vi "Arm Motor Control.vi"(6 "Left Arm EncoderDevRef":T1={"DevStatus"={"status"=FALSE, "code"=0, "source"=""}, "EncoderIndex"=enum."Invalid", "CounterIndex"=enum."Ctr 1", "DistancePerCount"=2.0, "Decoding Type"=enum."4x"}, 7 "Right Arm EncoderDevRef":T1={"DevStatus"={"status"=FALSE, "code"=0, "source"=""}, "EncoderIndex"=enum."Invalid", "CounterIndex"=enum."Ctr 1", "DistancePerCount"=2.0, "Decoding Type"=enum."4x"}, 8 "Right Arm MotorControlDevRef":T5={"DeviceStatus"={"status"=FALSE, "code"=0, "source"=""}, "Type"=enum."PWM", "PWM"={"PWM Channel"=enum."Invalid", "DeadBand"={"Name"="", "maxPositivePwm"=0, "minPositivePwm"=0, "centerPwm"=0, "maxNegativePwm"=0, "minNegativePwm"=0, "angularRange"=0}}, "CAN"={"Device Number"=0, "Control Mode"=enum."Percent VBus", "Semaphore"=refnum, "Max Vout"=12.0, "TalonSRX Control Mode"=enum."Percent VBus"}, "Invert"=FALSE}, 9 "Left Arm MotorControlDevRef":T5={"DeviceStatus"={"status"=FALSE, "code"=0, "source"=""}, "Type"=enum."PWM", "PWM"={"PWM Channel"=enum."Invalid", "DeadBand"={"Name"="", "maxPositivePwm"=0, "minPositivePwm"=0, "centerPwm"=0, "maxNegativePwm"=0, "minNegativePwm"=0, "angularRange"=0}}, "CAN"={"Device Number"=0, "Control Mode"=enum."Percent VBus", "Semaphore"=refnum, "Max Vout"=12.0, "TalonSRX Control Mode"=enum."Percent VBus"}, "Invert"=FALSE}) -> (0 "Left Arm EncoderDevRef":T1={"DevStatus"={"status"=FALSE, "code"=0, "source"=""}, "EncoderIndex"=enum."Invalid", "CounterIndex"=enum."Ctr 1", "DistancePerCount"=2.0, "Decoding Type"=enum."4x"}, 1 "Right Arm EncoderDevRef":T1={"DevStatus"={"status"=FALSE, "code"=0, "source"=""}, "EncoderIndex"=enum."Invalid", "CounterIndex"=enum."Ctr 1", "DistancePerCount"=2.0, "Decoding Type"=enum."4x"}, 2 "Right Arm MotorControlDevRef 2":T5={"DeviceStatus"={"status"=FALSE, "code"=0, "source"=""}, "Type"=enum."PWM", "PWM"={"PWM Channel"=enum."Invalid", "DeadBand"={"Name"="", "maxPositivePwm"=0, "minPositivePwm"=0, "centerPwm"=0, "maxNegativePwm"=0, "minNegativePwm"=0, "angularRange"=0}}, "CAN"={"Device Number"=0, "Control Mode"=enum."Percent VBus", "Semaphore"=refnum, "Max Vout"=12.0, "TalonSRX Control Mode"=enum."Percent VBus"}, "Invert"=FALSE}, 3 "Left Arm MotorControlDevRef 2":T5={"DeviceStatus"={"status"=FALSE, "code"=0, "source"=""}, "Type"=enum."PWM", "PWM"={"PWM Channel"=enum."Invalid", "DeadBand"={"Name"="", "maxPositivePwm"=0, "minPositivePwm"=0, "centerPwm"=0, "maxNegativePwm"=0, "minNegativePwm"=0, "angularRange"=0}}, "CAN"={"Device Number"=0, "Control Mode"=enum."Percent VBus", "Semaphore"=refnum, "Max Vout"=12.0, "TalonSRX Control Mode"=enum."Percent VBus"}, "Invert"=FALSE})   [LabVIEW 2015]
uses:
  <vilib>/Rock Robotics/WPI/MotorControl/WPI_MotorControlDeviceRef.ctl
  <vilib>/Rock Robotics/WPI/MotorControl/WPI_MotorControlType.ctl
  <vilib>/Rock Robotics/SystemInterfaces/DIO/FPGA_DIOPWMChannel.ctl
  <vilib>/Rock Robotics/WPI/PWM/WPI_PWMDeadband.ctl
  <vilib>/Rock Robotics/WPI/CAN/Jaguar/SubVIs/WPI_CANJaguar_ControlMode.ctl
  <vilib>/Rock Robotics/WPI/CAN/TalonSRX/WPI_CANTalonSRX_APIControlMode.ctl
  <vilib>/Rock Robotics/WPI/Encoder/WPI_EncoderDevRef.ctl
  <vilib>/Rock Robotics/SystemInterfaces/Encoder/FPGA_EncoderIdx.ctl
  <vilib>/Rock Robotics/SystemInterfaces/Counter/FPGA_CounterCtrSystemIndex.ctl
  <vilib>/Rock Robotics/WPI/Encoder/WPI_EncoderType.ctl
  Robot Values.vi
  <vilib>/addons/control/pid/NI_PID_pid.lvlib
  <vilib>/addons/control/pid/pid.llb/PID (DBL).vi
panel:
  in  "Initialize arm position":dbl=0.3 format="%#_13g"
  in  "Gravity Fighter":dbl=0.1 format="%#_13g"
  in  "Power Multiplier":dbl=0.5 format="%#_13g"
  out "output":bool
  in  "Right Arm PID gains":T12={"proportional gain (Kc)"=0.017, "integral time (Ti, min)"=0.0, "derivative time (Td, min)"=0.0} {"derivative time (Td, min)" format="%.3f"; "integral time (Ti, min)" format="%.3f"; "proportional gain (Kc)" format="%.3f"}
  in  "Left Arm PID gains":T12={"proportional gain (Kc)"=0.017, "integral time (Ti, min)"=0.0, "derivative time (Td, min)"=0.0} {"derivative time (Td, min)" format="%.3f"; "integral time (Ti, min)" format="%.3f"; "proportional gain (Kc)" format="%.3f"}
  # "For no Load: \nP:.003\nI: .010\nD: .000"
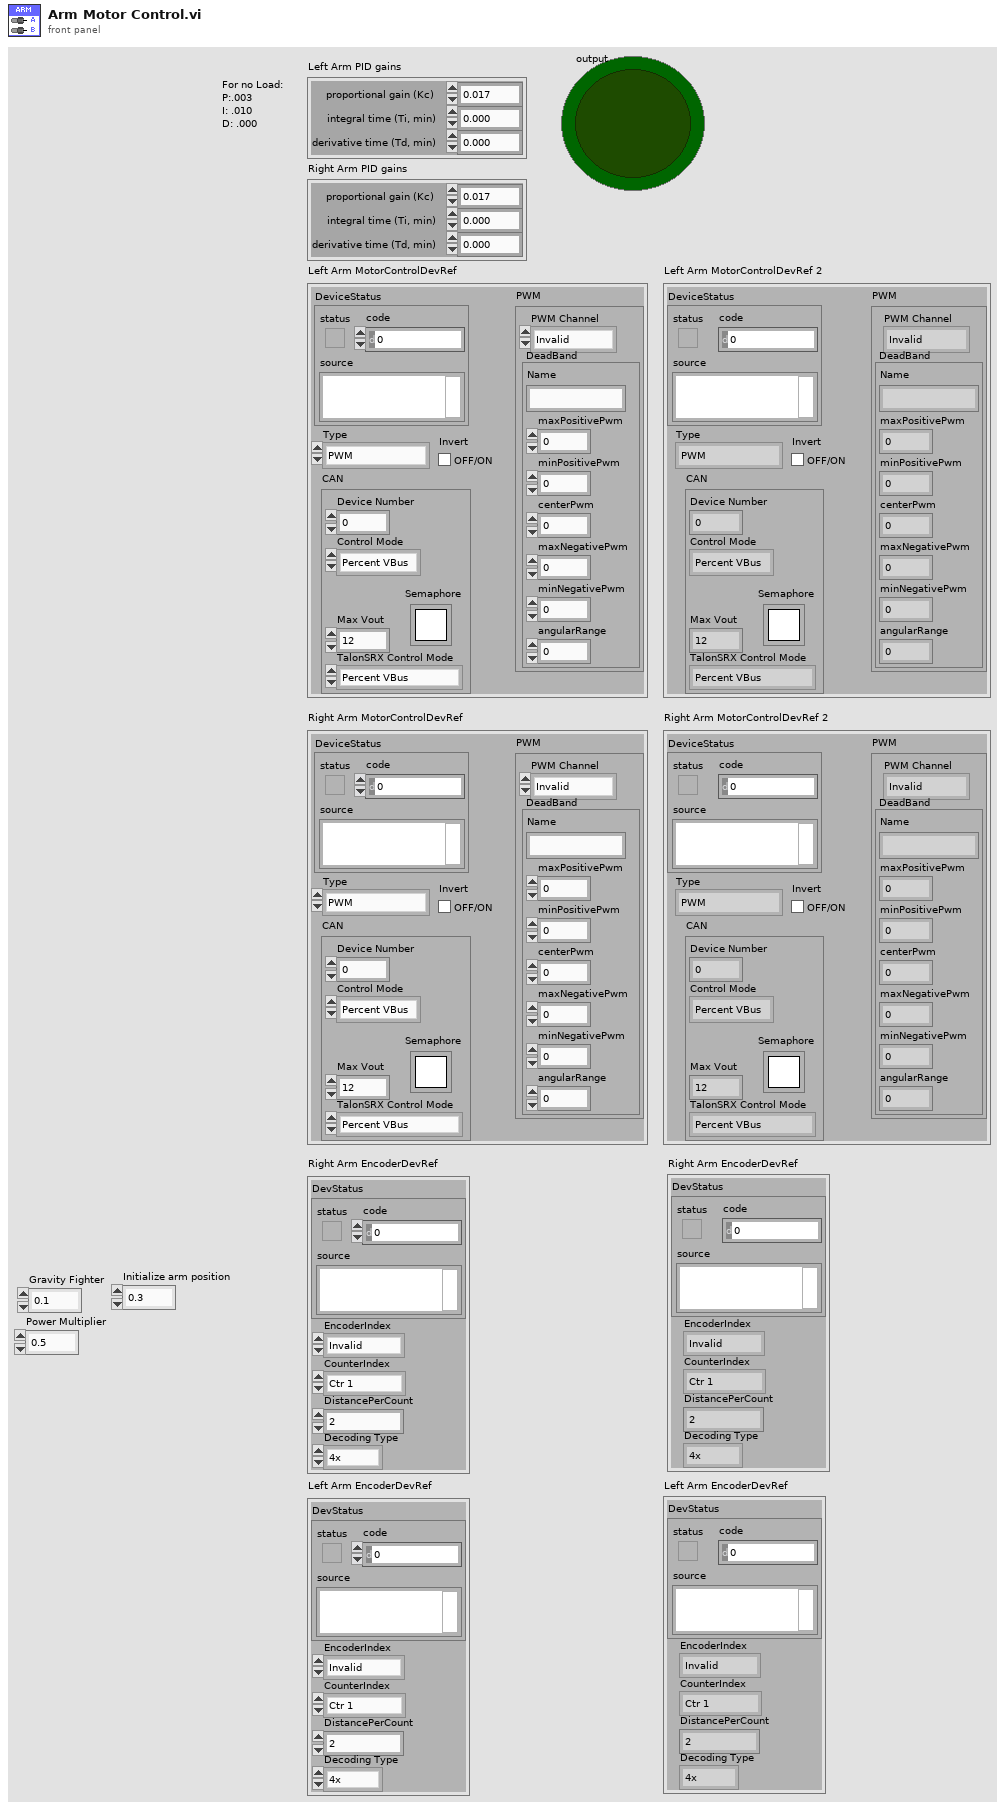
[diagram p1: front panel]
types:
  T1 = typedef "WPI_EncoderDevRef.ctl" = cluster{"DevStatus":errorcluster, "EncoderIndex":T2, "CounterIndex":T3, "DistancePerCount":dbl, "Decoding Type":T4}
  T2 = typedef "FPGA_EncoderIdx.ctl" = enum8{"Enc 0", "Enc 1", "Enc 2", "Enc 3", "Enc 4", "Enc 5", "Enc 6", "Enc 7", "Invalid"}
  T3 = typedef "FPGA_CounterCtrSystemIndex.ctl" = enum8{"Ctr 0", "Ctr 1", "Ctr 2", "Ctr 3", "Ctr 4", "Ctr 5", "Ctr 6", "Ctr 7", "Invalid"}
  T4 = typedef "WPI_EncoderType.ctl" = enum16{"1x", "2x", "4x"}
  T5 = typedef "WPI_MotorControlDeviceRef.ctl" = cluster{"DeviceStatus":errorcluster, "Type":T6, "PWM":cluster{"PWM Channel":T7, "DeadBand":T8}, "CAN":cluster{"Device Number":u8, "Control Mode":T9, "Semaphore":T10, "Max Vout":dbl, "TalonSRX Control Mode":T11}, "Invert":bool}
  T6 = typedef "WPI_MotorControlType.ctl" = enum16{"PWM", "CAN", "CANTalonSRX"}
  T7 = typedef "FPGA_DIOPWMChannel.ctl" = enum8{"PWM 0", "PWM 1", "PWM 2", "PWM 3", "PWM 4", "PWM 5", "PWM 6", "PWM 7", "PWM 8", "PWM 9", "PWM MXP 0", "PWM MXP 1", "PWM MXP 2", "PWM MXP 3", "PWM MXP 4", "PWM MXP 5", "PWM MXP 6", "PWM MXP 7", "PWM MXP 8", "PWM MXP 9", "Invalid"}
  T8 = typedef "WPI_PWMDeadband.ctl" = cluster{"Name":string, "maxPositivePwm":i32, "minPositivePwm":i32, "centerPwm":i32, "maxNegativePwm":i32, "minNegativePwm":i32, "angularRange":u16}
  T9 = typedef "WPI_CANJaguar_ControlMode.ctl" = enum8{"Percent VBus", "Current", "Speed", "Position", "Voltage"}
  T10 = typedef "Semaphore RefNum" = refnum<k1>
  T11 = typedef "WPI_CANTalonSRX_APIControlMode.ctl" = enum8{"Percent VBus", "Speed", "Position", "Slave", "Unchanged / Invalid", "Voltage Compensation", "Current", "Motion Profile"}
  T12 = cluster{"proportional gain (Kc)":dbl, "integral time (Ti, min)":dbl, "derivative time (Td, min)":dbl}
  T13 = typedef "Robot Values.ctl" = cluster{"Drive Motors":cluster{"Left Motor Value":dbl, "Right Motor Value":dbl, "Left Motor Encoder":dbl, "Right Motor Encoder":dbl, "High/Low Gear":bool}, "Sensors":cluster{"Gyro Angle":dbl, "Photoeye":bool, "Ultrasonic Range":dbl, "Shooter Speed Encoder":dbl, "Accelerometer Value":dbl, "Flashlight":bool, "Target Distance":dbl, "Target X Value":dbl, "Reset Gyro?":bool}, "Arms":cluster{"Desired Arm Position":dbl, "Left Arm Encoder":dbl, "Right Arm Encoder":dbl, "Left Arm Lower Limit":bool, "Right Arm Lower Limit":bool, "Initialize Arm Position?":bool}, "Acquisition and Scoring":cluster{"Acquiring?":bool, "Current Speed":dbl, "Setpoint Speed":dbl, "Prep Wheels":bool, "Shoot":bool, "Low Eject":bool, "Reverse Shooter Wheel":bool}, "Hanging":cluster{"Pivot Arms":dbl, "PTO":bool, "Left Pivot Encoder":dbl, "Right Pivot Encoder":dbl, "Hanging Pin":bool}}
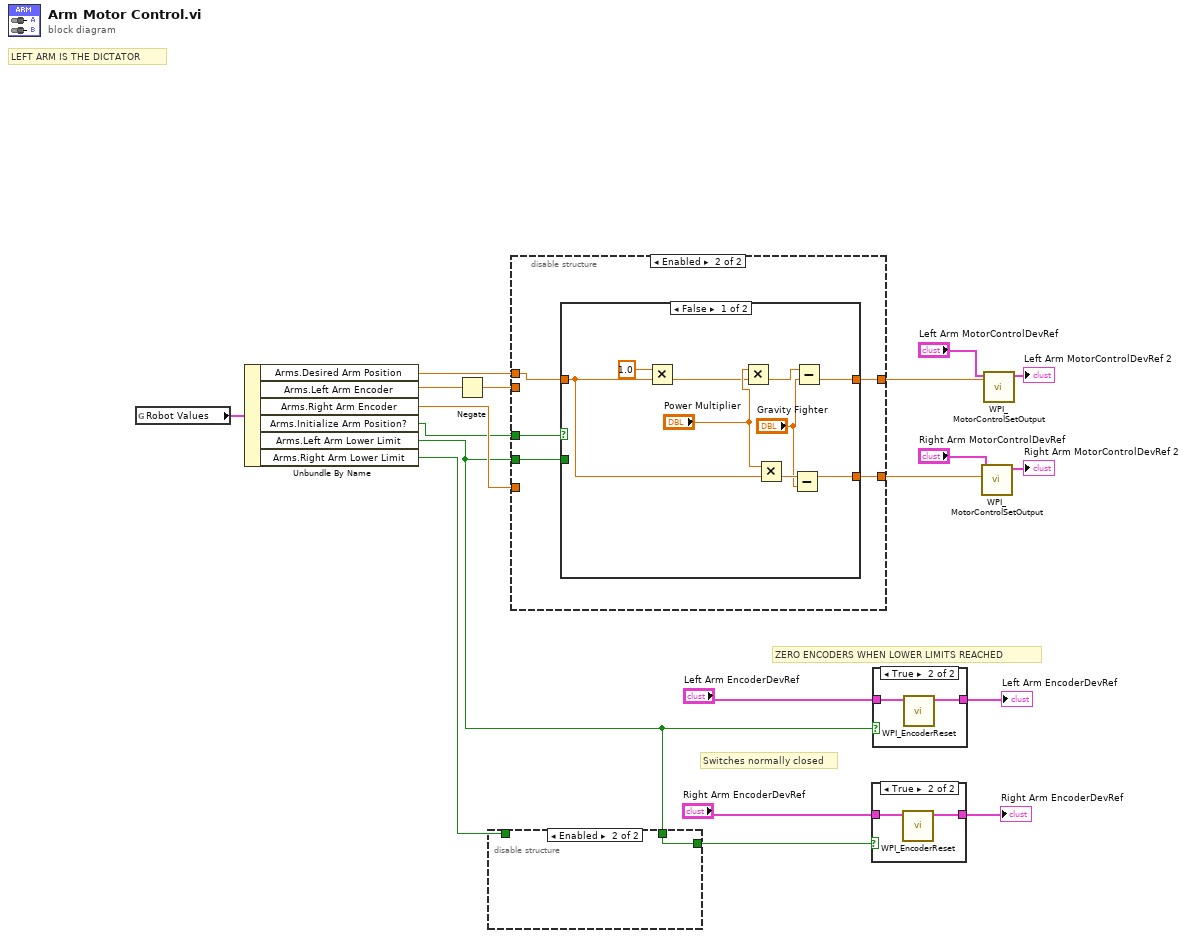
[diagram p0: block diagram]
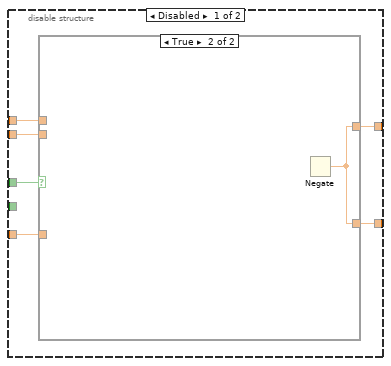
[diagram p2: hidden frame]
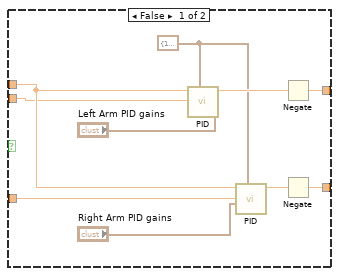
[diagram p3: hidden frame]
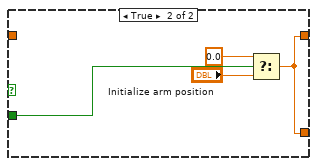
[diagram p4: hidden frame]
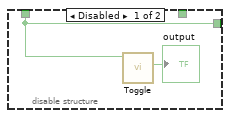
[diagram p5: hidden frame]
diagram:
  # "ZERO ENCODERS WHEN LOWER LIMITS REACHED"
  # "Switches normally closed"
  # "LEFT ARM IS THE DICTATOR"
  n1 = global read "Robot Values.vi" "Robot Values"() -> (w17:T13)
  n2 = Unbundle By Name(w17) -> ("Arms.Desired Arm Position"=w14:dbl, "Arms.Left Arm Encoder"=w19:dbl, "Arms.Right Arm Encoder"=w18:dbl, "Arms.Initialize Arm Position?"=w2:bool, "Arms.Left Arm Lower Limit"=w1:bool, "Arms.Right Arm Lower Limit"=w9:bool)
  n3 = Negate(x=w19) -> (-x=w8:dbl)
  n4 = disable-structure shown="Enabled" {
    disable-tunnel: w9 -> [w21 _]
    disable-tunnel: [w21 w22] -> w7
    disable-tunnel: w1 -> [_ w22]
    frame Disabled {
      n5 = call "Toggle.vi"("Input"=w21) -> ("output"=→"output":bool)  [unwired: 10 in]
    }
    frame Enabled {
    }
  }
  n6 = disable-structure shown="Enabled" {
    disable-tunnel: w18 -> [w28 _]
    disable-tunnel: [w27 w43] -> w16
    disable-tunnel: [w26 w42] -> w15
    disable-tunnel: w14 -> [w25 w44]
    disable-tunnel: w8 -> [w24 _]
    disable-tunnel: w2 -> [w23 w41]
    disable-tunnel: w1 -> [_ w40]
    frame Disabled {
      n7 = case shown="True" w23 {
        tunnel: w28 -> [w38 _]
        tunnel: [w37 w39] -> w27
        tunnel: [w36 w39] -> w26
        tunnel: w25 -> [w35 _]
        tunnel: w24 -> [w34 _]
        frame False {
          w29 = cluster{"output high":dbl, "output low":dbl} {"output high"=1.0, "output low"=-1.0} ("output range")
          n8 = call-poly <vilib>:"PID.vi"("output range"=w29, "PID gains"="Left Arm PID gains", "process variable"=w34, "setpoint"=w35) -> ("output"=w33:dbl)  [unwired: 6 in, 1 out]
          n9 = call-poly <vilib>:"PID.vi"("output range"=w29, "PID gains"="Right Arm PID gains", "process variable"=w38, "setpoint"=w35) -> ("output"=w31:dbl)  [unwired: 6 in, 1 out]
          n10 = Negate(x=w33) -> (-x=w37:dbl)
          n11 = Negate(x=w31) -> (-x=w36:dbl)
        }
        frame True {
          n12 = Negate() -> (-x=w39:dbl)  [unwired: 1 in]
        }
      }
    }
    frame Enabled {
      n13 = case shown="False" w41 {
        tunnel: w44 -> [w53 _]
        tunnel: [w50 w54] -> w43
        tunnel: [w49 w54] -> w42
        tunnel: w40 -> [_ w57]
        frame False {
          n14 = Multiply(x=1.0, y=w53) -> (x*y=w46:dbl)
          n15 = Multiply(x="Power Multiplier", y=w46) -> (x*y=w48:dbl)
          n16 = Multiply(x="Power Multiplier", y=w53) -> (x*y=w52:dbl)
          n17 = Subtract(x=w52, y="Gravity Fighter") -> (x-y=w49:dbl)
          n18 = Subtract(x=w48, y="Gravity Fighter") -> (x-y=w50:dbl)
        }
        frame True {
          n19 = Select(t=0.0, s=w57, f="Initialize arm position") -> (s? t:f=w54:dbl)
        }
      }
    }
  }
  n20 = case shown="True" w7 {
    tunnel: "Right Arm EncoderDevRef" -> [w58 w60]
    tunnel: [w58 w59] -> w10
    frame False {
    }
    frame True {
      n21 = call <vilib>:"WPI_EncoderReset.vi"("EncoderDevRef"=w60) -> ("EncoderDevRef"=w59:T1)  [unwired: 9 in, 1 out]
    }
  }
  "Right Arm EncoderDevRef" <- w10
  n22 = case shown="True" w1 {
    tunnel: "Left Arm EncoderDevRef" -> [w61 w63]
    tunnel: [w61 w62] -> w12
    frame False {
    }
    frame True {
      n23 = call <vilib>:"WPI_EncoderReset.vi"("EncoderDevRef"=w63) -> ("EncoderDevRef"=w62:T1)  [unwired: 9 in, 1 out]
    }
  }
  "Left Arm EncoderDevRef" <- w12
  n24 = call <vilib>:"WPI_MotorControlSetOutput.vi"("Output"=w15, "MotorControlDevRef"="Right Arm MotorControlDevRef") -> ("MotorControlDevRef"=→"Right Arm MotorControlDevRef 2":T5)  [unwired: 7 in, 2 out]
  n25 = call <vilib>:"WPI_MotorControlSetOutput.vi"("Output"=w16, "MotorControlDevRef"="Left Arm MotorControlDevRef") -> ("MotorControlDevRef"=→"Left Arm MotorControlDevRef 2":T5)  [unwired: 7 in, 2 out]
